vi "Add New Node.vi"(6 "New Node Types":T1, 7 "Group Name":string, 8 "Default Element Value":string, 9 "Type Name":string, 10 "Text Nodes":cluster{"Name":string, "Value":string}[](array[cluster]), 11 "Doc Ref":refnum<k20>) -> (2 "Updated Node Ref":refnum<k20>)   [LabVIEW 2025]
uses:
  <resource>/objmgr/DOMUserDefRef.rc
  Types/New Node Types.ctl
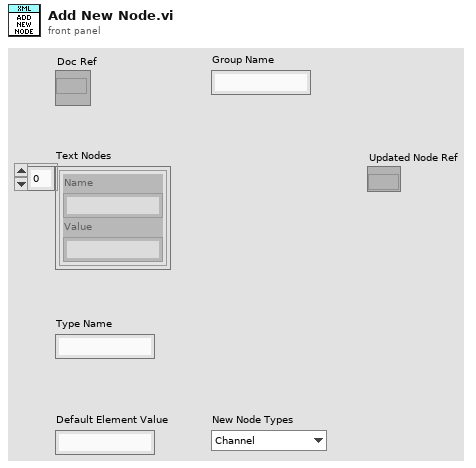
[diagram p1: front panel]
types:
  T1 = typedef "New Node Types.ctl" = enum16{"Channel", "Waveform", "Section"}
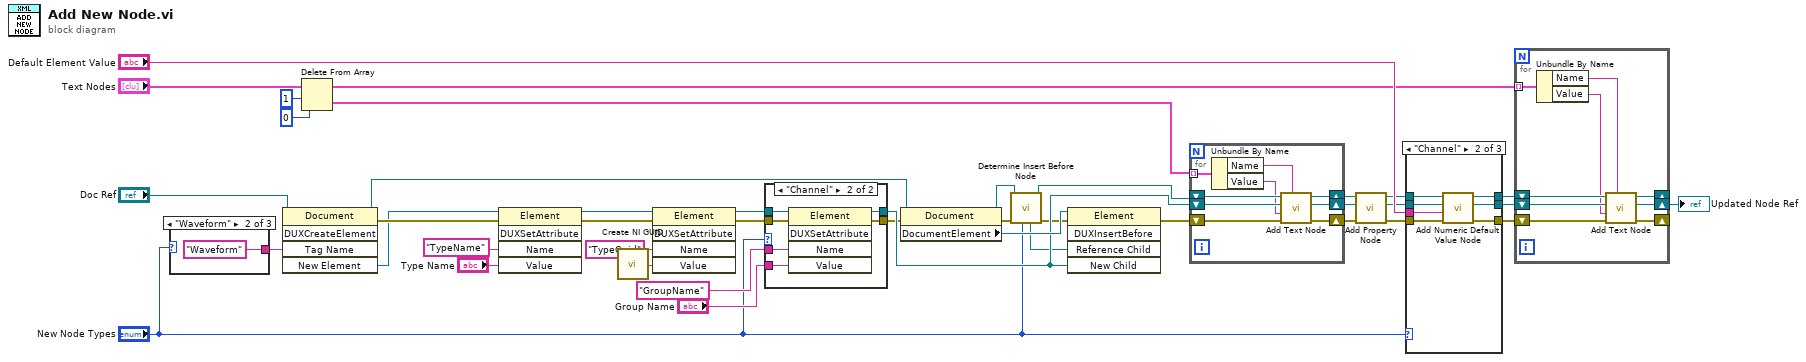
[diagram p0: block diagram]
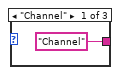
[diagram p3: hidden frame]
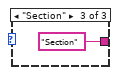
[diagram p4: hidden frame]
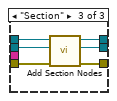
[diagram p6: hidden frame]
diagram:
  n1 = case shown="\"Waveform\"" "New Node Types" {
    tunnel: ["Channel" ("Tag Name") "Waveform" ("Tag Name") "Section" ("Tag Name")] -> w28
    frame "Channel" {
    }
    frame "Waveform" {
    }
    frame "Section" {
    }
  }
  n2 = invoke class="Document" method="DUXCreateElement"(reference="Doc Ref", "Tag Name"=w28) -> (reference out=w30:refnum<k20>, error out=w41:errorcluster, "New Element"=w33:refnum<k20>)  [unwired: 3 in, 2 out]
  n3 = Delete From Array(array="Text Nodes", length=1, index=0) -> (deleted portion=w17:cluster{"Name":string, "Value":string}[], array with subset deleted=w24:cluster{"Name":string, "Value":string}[])
  n4 = invoke class="Element" method="DUXSetAttribute"(reference=w33, error in=w41, "Name"="TypeName", "Value"="Type Name") -> (reference out=w32:refnum<k20>, error out=w35:errorcluster)  [unwired: 1 in, 3 out]
  n5 = call <vilib>:"Create NI GUID.vi"() -> ("NI GUID"=w38:string)
  n6 = invoke class="Element" method="DUXSetAttribute"(reference=w32, error in=w35, "Name"="TypeGuid", "Value"=w38) -> (reference out=w8:refnum<k20>, error out=w10:errorcluster)  [unwired: 1 in, 3 out]
  n7 = case shown="\"Channel\"" "New Node Types" {
    tunnel: w10 -> [w45 w52]
    tunnel: [w45 w51] -> w9
    tunnel: w8 -> [w46 w50]
    tunnel: [w46 w49] -> w19
    tunnel: "GroupName" ("Name") -> [_ w48]
    tunnel: "Group Name" -> [_ w47]
    frame Default {
    }
    frame "Channel" {
      n8 = invoke class="Element" method="DUXSetAttribute"(reference=w50, error in=w52, "Name"=w48, "Value"=w47) -> (reference out=w49:refnum<k20>, error out=w51:errorcluster)  [unwired: 1 in, 3 out]
    }
  }
  n9 = property class="Document"(reference=w30, error in=w9) -> (reference out=w29:refnum<k20>, error out=w31:errorcluster, "DocumentElement"=w34:refnum<k20>)
  n10 = call "Determine Insert Before Node.vi"("New Node"="New Node Types", "error in"=w31, "Document in"=w29) -> ("error out"=w4:errorcluster, "Document out"=w18:refnum<k20>, "Insert Before Node"=w3:refnum<k20>)  [unwired: 6 in]
  n11 = invoke class="Element" method="DUXInsertBefore"(reference=w34, error in=w4, "Reference Child"=w3, "New Child"=w19) -> (error out=w23:errorcluster)  [unwired: 1 in, 4 out]
  n12 = for {
    tunnel: w17 -> [w55] mode=indexing
    shift-right: [w61] -> w22
    shift-left: w23 -> [w60]
    shift-right: [w56] -> w20
    shift-left: w18 -> [w57]
    shift-right: [w58] -> w21
    shift-left: w19 -> [w59]
    n13 = Unbundle By Name(w55) -> ("Name"=w54:string, "Value"=w53:string)
    n14 = call "Add Text Node.vi"("Tag Name"=w54, "error in"=w60, "Tag Data"=w53, "Element in"=w59, "Document in"=w57) -> ("error out"=w61:errorcluster, "Element out"=w58:refnum<k20>, "Document out"=w56:refnum<k20>)  [unwired: 4 in]
  }
  n15 = call "Add Property Node.vi"("error in"=w22, "Element in"=w21, "Document in"=w20) -> ("error out"=w16:errorcluster, "Element out"=w14:refnum<k20>, "Document out"=w15:refnum<k20>)  [unwired: 6 in]
  n16 = case shown="\"Channel\"" "New Node Types" {
    tunnel: "Default Element Value" -> [_ w71 _]
    tunnel: w16 -> [w63 w70 w74]
    tunnel: w15 -> [w64 w69 w77]
    tunnel: w14 -> [w62 w68 w75]
    tunnel: [w64 w67 w76] -> w11
    tunnel: [w63 w66 w73] -> w13
    tunnel: [w62 w65 w72] -> w12
    frame Default {
    }
    frame "Channel" {
      n17 = call "Add Numeric Default Value Node.vi"("error in"=w70, "Default Value"=w71, "Element in"=w68, "Document in"=w69) -> ("error out"=w66:errorcluster, "Element out"=w65:refnum<k20>, "Document out"=w67:refnum<k20>)  [unwired: 5 in]
    }
    frame "Section" {
      n18 = call "Add Section Nodes.vi"("error in"=w74, "DOM Element in"=w75, "DOM document in"=w77) -> ("error out"=w73:errorcluster, "Document Element out"=w72:refnum<k20>, "DOM document out"=w76:refnum<k20>)  [unwired: 6 in]
    }
  }
  n19 = for {
    tunnel: w24 -> [w80] mode=indexing
    shift-right: [w86] -> _
    shift-left: w13 -> [w85]
    shift-right: [w81] -> _
    shift-left: w11 -> [w82]
    shift-right: [w83] -> w1
    shift-left: w12 -> [w84]
    n20 = Unbundle By Name(w80) -> ("Name"=w79:string, "Value"=w78:string)
    n21 = call "Add Text Node.vi"("Tag Name"=w79, "error in"=w85, "Tag Data"=w78, "Element in"=w84, "Document in"=w82) -> ("error out"=w86:errorcluster, "Element out"=w83:refnum<k20>, "Document out"=w81:refnum<k20>)  [unwired: 4 in]
  }
  "Updated Node Ref" <- w1
